vi "test_set_and_read_int64.vi"() -> ()   [LabVIEW 2019, in "Picam.lvclass"]
uses:
  Picam.lvclass
  picam32_LabView_SDK/PICam_lib/types/PicamModel.ctl
panel:
  in  "Accumulations set":i64=10
  out "Accumulations get":i64
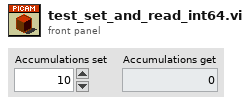
[diagram p1: front panel]
types:
  T1 = typedef "PicamModel.ctl" = u32
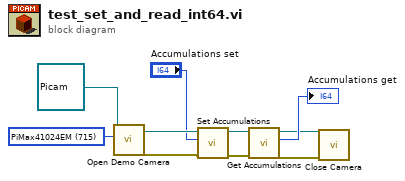
[diagram p0: block diagram]
diagram:
  w2 = T1 715 items=["---PIXIS 100 SERIES---"=1000, "PixisSeries"=0, "Pixis100BR"=5, "---PI-MAX4 SERIES---"=1001, "Pimax4Series"=700, "PiMax41024EM"=715] ("PicamModel")
  n1 = call-dynamic "Open Demo Camera.vi"("PicamModel"=w2, "Picam in"=refnum<class "Picam.lvclass"> refnum) -> ("error out"=w10:errorcluster, "Picam out"=w9:refnum<class "Picam.lvclass">)  [unwired: 8 in]
  n2 = call-dynamic "Set Accumulations.vi"("error in (no error)"=w10, "Accumulations"="Accumulations set", "Picam in"=w9) -> ("error out"=w7:errorcluster, "Picam out"=w6:refnum<class "Picam.lvclass">)  [unwired: 7 in]
  n3 = call-dynamic "Get Accumulations.vi"("error in (no error)"=w7, "Picam in"=w6) -> ("error out"=w4:errorcluster, "Accumulations"=→"Accumulations get":i64, "Picam out"=w3:refnum<class "Picam.lvclass">)  [unwired: 7 in]
  n4 = call-dynamic "Close Camera.vi"("error in (no error)"=w4, "Picam in"=w3) -> ()  [unwired: 8 in, 2 out]
